vi "Read OPCUA.lvclass.vi"(8 "error in (no error)":errorcluster, 11 "Model_AMC in":refnum<class "Model_AMC.lvclass">) -> (0 "error out":errorcluster, 2 "OPCUA.lvlib:OPCUA.lvclass":refnum<class "OPCUA.lvclass">, 3 "Model_AMC out":refnum<class "Model_AMC.lvclass">)   [LabVIEW 2021, in "Model_AMC.lvclass"]
uses:
  Model_AMC.lvclass
  Model_AMC.lvclass/Model_AMC.ctl
  <userlib>/John_Lib/OPCUA/OPCUA.lvclass
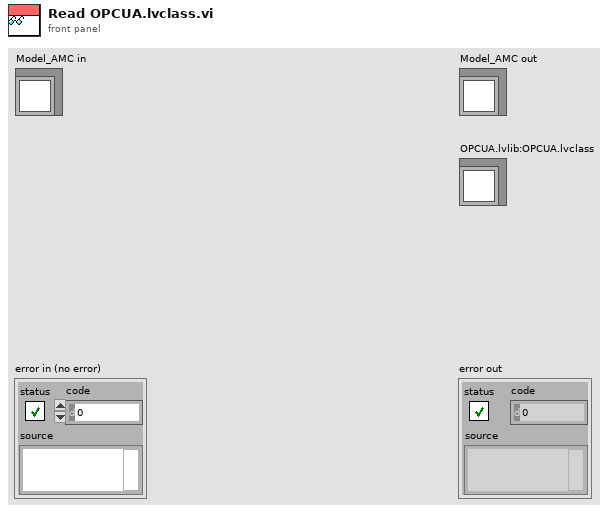
[diagram p1: front panel]
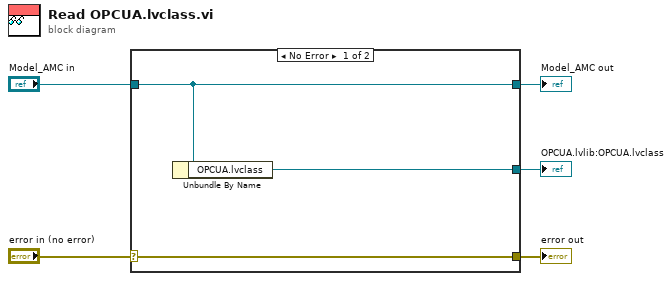
[diagram p0: block diagram]
diagram:
  n1 = case shown="No Error" "error in (no error)" {
    selector: "error in (no error)" -> [w8 w9]
    tunnel: [w8 w9] -> w4
    tunnel: [w7 w10] -> w2
    tunnel: "Model_AMC in" -> [w7 w10]
    tunnel: [w6 _] -> w1
    frame No Error {
      n2 = Unbundle By Name(w7) -> ("OPCUA.lvclass"=w6:refnum<class "OPCUA.lvclass">)
    }
    frame Error {
    }
  }
  "error out" <- w4
  "Model_AMC out" <- w2
  "OPCUA.lvlib:OPCUA.lvclass" <- w1
